vi "Set Control Font.vi"(4 "Error In":errorcluster, 6 "Font Parameters":T1, 7 "Font Settting in":refnum<class "Display Properties.lvclass">) -> (0 "Error Out":errorcluster, 3 "Font Settting out":refnum<class "Display Properties.lvclass">)   [LabVIEW 2015, in "Display Properties Manager.lvlib" / "Display Properties.lvclass"]
uses:
  Display Properties.lvclass
  _typedefs/Font Parameters.ctl
  _typedefs/Control Component to Set.ctl
  Display Properties.lvclass/Display Properties.ctl
  Display Properties Manager.lvlib
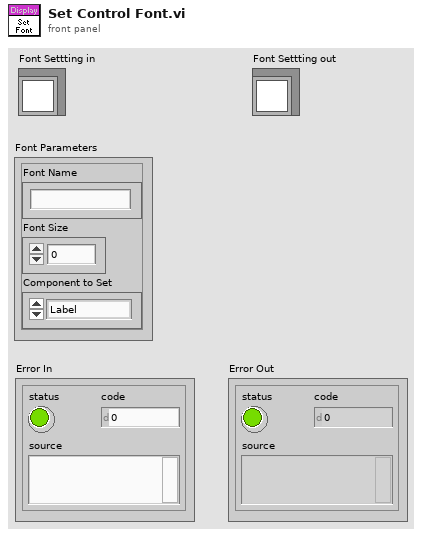
[diagram p1: front panel]
types:
  T1 = typedef "Display Properties Manager.lvlib/Font Parameters.ctl" = cluster{"Font Name":string, "Font Size":u32, "Component to Set":T2}
  T2 = typedef "Display Properties Manager.lvlib/Control Component to Set.ctl" = enum16{"Label", "Caption", "Contents"}
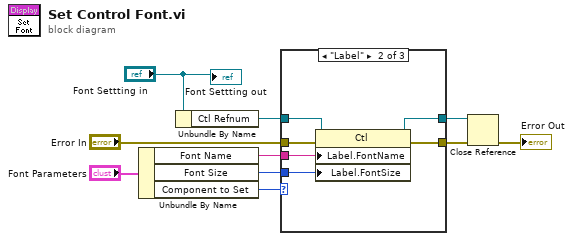
[diagram p0: block diagram]
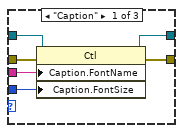
[diagram p2: hidden frame]
diagram:
  n1 = Unbundle By Name("Font Parameters") -> ("Font Name"=w6:string, "Font Size"=w5:u32, "Component to Set"=w4:T2)
  n2 = Unbundle By Name("Font Settting in") -> ("Ctl Refnum"=w1:refnum<vi>)
  n3 = case shown="\"Label\"" w4 {
    tunnel: [w16 w22 w23] -> w9
    tunnel: [w15 w21 w24] -> w8
    tunnel: "Error In" -> [w14 w19 w23]
    tunnel: w1 -> [w13 w20 w24]
    tunnel: w6 -> [w12 w18 _]
    tunnel: w5 -> [w11 w17 _]
    frame "Caption" {
      n4 = property class="Ctl"(reference=w13, error in=w14, "Caption.FontName"=w12, "Caption.FontSize"=w11) -> (reference out=w15:refnum<vi>, error out=w16:errorcluster)
    }
    frame "Label" {
      n5 = property class="Ctl"(reference=w20, error in=w19, "Label.FontName"=w18, "Label.FontSize"=w17) -> (reference out=w21:refnum<vi>, error out=w22:errorcluster)
    }
    frame "Contents" {
    }
  }
  n6 = Close Reference(reference=w8, error in (no error)=w9) -> (error out=→"Error Out":errorcluster)
  "Font Settting out" <- "Font Settting in"
